vi "Modulator.vi"(8 "error in (no error)":errorcluster, 11 "ISO 14443 A UP in":refnum<class "ISO 14443 A UP.lvclass">) -> (0 "error out":errorcluster, 2 "Waveform out":waveform(dbl), 3 "ISO 14443 A UP out":refnum<class "ISO 14443 A UP.lvclass">)   [LabVIEW 2019, in "ISO 14443 A UP.lvclass"]
uses:
  ISO 14443 A UP.lvclass
  TypeDef/Store.ctl
  ISO 14443 A UP.lvclass/ISO 14443 A UP.ctl
  <vilib>/addons/Modulation/Analog/MT Modulate AM (DSB).vi
  <vilib>/addons/Modulation/Analog/MT Upconvert Baseband (Real).vi
  <vilib>/addons/Modulation/niAMT.lvlib
  RFID system.lvclass
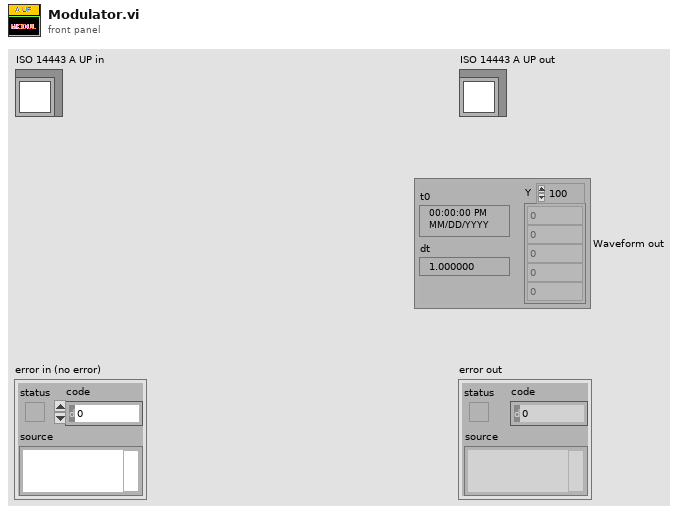
[diagram p1: front panel]
types:
  T1 = typedef "Store.ctl" = enum16{"envelope", "noise", "demSubCar", "CH_frame", "Decode", "demodulate", "in", "out", "sum", "subCarrier", "frame", "command", "encode", "modulate", "encode_UP", "modulate_up", "demod_up", "envelop_up", "sum_up", "out_up", "in_up"}
  T2 = typedef "niAMT.lvlib/Complex Data Waveform.ctl" = cluster{"t0":dbl, "dt":dbl, "Y":cdb[]}
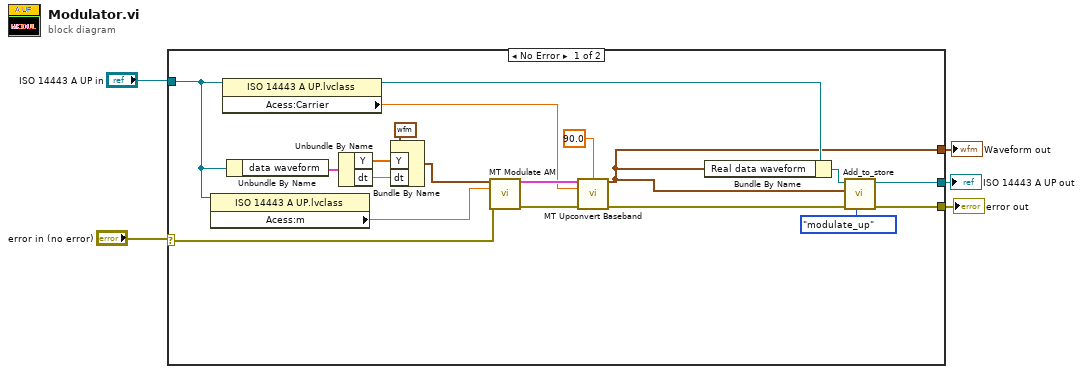
[diagram p0: block diagram]
diagram:
  n1 = case shown="No Error" "error in (no error)" {
    selector: "error in (no error)" -> [w15 w25]
    tunnel: "ISO 14443 A UP in" -> [w8 w26]
    tunnel: [w11 w26] -> w2
    tunnel: [w10 w25] -> w3
    tunnel: [w6 _] -> w1
    frame No Error {
      n2 = property class="ISO 14443 A UP.lvclass"(reference=w8) -> ("Acess:m"=w7:dbl)  [unwired: 1 in, 2 out]
      n3 = property class="ISO 14443 A UP.lvclass"(reference=w8) -> (reference out=w14:refnum<class "ISO 14443 A UP.lvclass">, "Acess:Carrier"=w16:dbl)  [unwired: 1 in, 1 out]
      n4 = Unbundle By Name(w8) -> ("data waveform"=w17:T2)
      n5 = Unbundle By Name(w17) -> ("Y"=w19:cdb[], "dt"=w18:dbl)
      n6 = Bundle By Name(cluster=waveform(cdb) {"t0"=timestamp(0 s since 1904-01-01), "dt"=1.0, "Y"=[]} ("waveform"), "Y"=w19, "dt"=w18) -> (w21:waveform(cdb))
      n7 = call-poly <vilib>:"MT Modulate AM.vi"("message signal"=w21, "modulation index"=w7, "error in (no error)"=w15) -> ("AM modulated waveform"=w20:cluster{"t0":dbl, "dt":dbl, "Y":cdb[]}, "error out"=w23:errorcluster)  [unwired: 11 in]
      n8 = call-poly <vilib>:"MT Upconvert Baseband.vi"("baseband waveform (complex)"=w20, "initial phase (deg)"=90.0, "carrier frequency (Hz)"=w16, "error in (no error)"=w23) -> ("passband waveform"=w6:waveform(dbl), "error out"=w12:errorcluster)  [unwired: 10 in]
      n9 = Bundle By Name(cluster=w14, "Real data waveform"=w6) -> (w13:refnum<class "ISO 14443 A UP.lvclass">)
      n10 = call "Add_to_store.vi"("Store"=Store."modulate_up", "error in (no error)"=w12, "Waveform"=w6, "RFID system in"=w13) -> ("error out"=w10:errorcluster, "RFID system out"=w11:refnum<class "ISO 14443 A UP.lvclass">)  [unwired: 6 in]
    }
    frame Error {
    }
  }
  "error out" <- w3
  "ISO 14443 A UP out" <- w2
  "Waveform out" <- w1
